vi "Coverate Include File Path From Test Cases.vi"(11 "Test Case Classes":path[](array[path])) -> (3 "appended path":path)   [LabVIEW 2020, in "Coverage Report.lvclass"]
uses:
  Coverage Report.lvclass
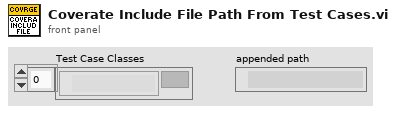
[diagram p1: front panel]
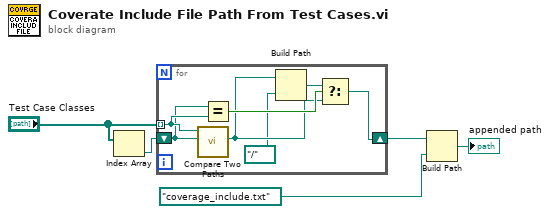
[diagram p0: block diagram]
diagram:
  n1 = Index Array(array="Test Case Classes") -> (element=w2:path)  [unwired: 1 in]
  n2 = for {
    tunnel: "Test Case Classes" -> [w12] mode=indexing
    shift-right: [w9] -> w3
    shift-left: w2 -> [w11]
    n3 = call <vilib>:"Compare Two Paths.vi"("Path 2"=w11, "Path 1"=w12) -> ("Common Path"=w7:path)  [unwired: 6 in, 3 out]
    n4 = Equal?(x=w11, y=w12) -> (x = y?=w10:bool)
    n5 = Build Path(base path=w7, name or relative path=path "../..") -> (appended path=w8:path)
    n6 = Select(t=w8, s=w10, f=w7) -> (s? t:f=w9:path)
  }
  n7 = Build Path(base path=w3, name or relative path=path "coverage_include.txt") -> (appended path=→"appended path":path)
